vi "DAQ_Initialization.vi"(4 "AO Lasers":tag="USB-6363/ao0:3", 5 "AO Z":tag="USB-6211/ao1", 6 "AO Pockels":tag="USB-6211/ao0", 7 "DO":tag="USB-6363/port0/line0:3", 8 "error in (no error)":errorcluster, 9 "Counter":tag="USB-6363/ctr0", 10 "Timing source":tag="OnboardClock", 11 "DO | Trigger":tag="/USB-6363/PFI12") -> (0 "error out":errorcluster)   [LabVIEW 2025]
uses:
  <vilib>/DAQmx/create/channels.llb/DAQmx Create Channel (CO-Pulse Generation-Time).vi
  <vilib>/DAQmx/configure/events/hardwareSignals.llb/DAQmx Export Signal (Most Signals).vi
  <vilib>/DAQmx/create/channels.llb/DAQmx Create Channel (DO-Digital Output).vi
  <vilib>/DAQmx/configure/timing.llb/DAQmx Timing (Sample Clock).vi
  <vilib>/DAQmx/configure/trigger.llb/DAQmx Start Trigger (Digital Edge).vi
  <vilib>/DAQmx/create/channels.llb/DAQmx Create Channel (AO-Voltage-Basic).vi
  <resource>/objmgr/daqmx.rc
panel:
  in  "Export_Clock":tag="/USB-6211/PFI7"
  in  "Export_Trigger":tag="/USB-6363/PFI12"
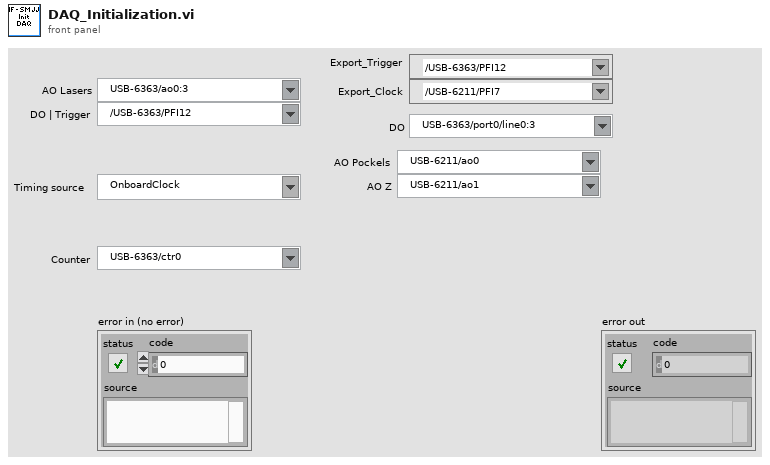
[diagram p1: front panel]
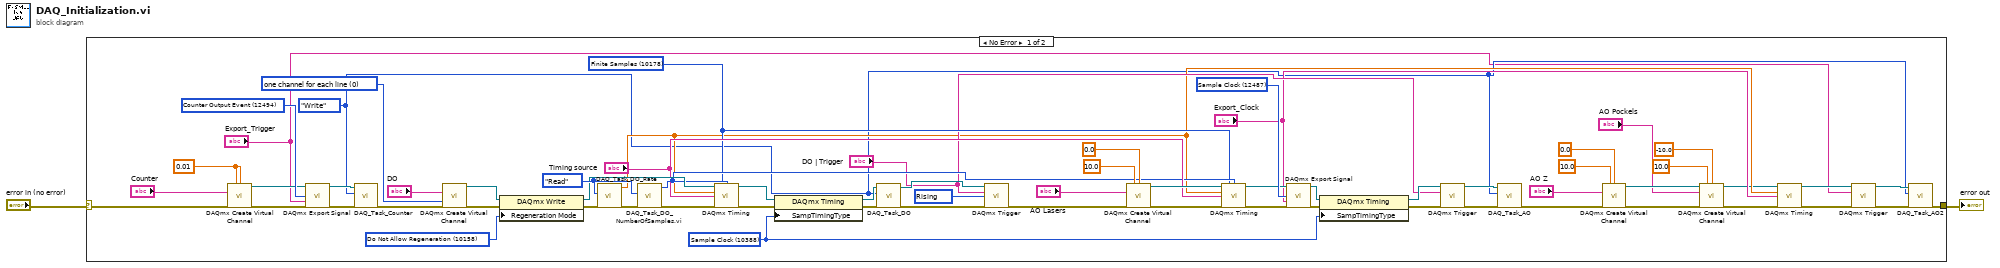
[diagram p0: block diagram]
diagram:
  n1 = case shown="No Error" "error in (no error)" {
    selector: "error in (no error)" -> [w48 w69]
    tunnel: [w12 w69] -> w1
    frame No Error {
      w25 = 12487 items=["AI Convert Clock"=12484, "10MHz Reference Clock"=12536, "20MHz Timebase Clock"=12486, "Sample Clock"=12487, "Advance Trigger"=12488, "Reference Trigger"=12490, "Start Trigger"=12491, "Advance Complete Event"=12492, "AI Hold Complete Event"=12493, "Counter Output Event"=12494, "Change Detection Event"=12511, "Watchdog Timer Expired Event"=12512] ("signal")
      w30 = 12494 items=["AI Convert Clock"=12484, "10MHz Reference Clock"=12536, "20MHz Timebase Clock"=12486, "Sample Clock"=12487, "Advance Trigger"=12488, "Reference Trigger"=12490, "Start Trigger"=12491, "Advance Complete Event"=12492, "AI Hold Complete Event"=12493, "Counter Output Event"=12494, "Change Detection Event"=12511, "Watchdog Timer Expired Event"=12512] ("signal")
      w68 = 0 items=["one channel for each line", "one channel for all lines"] ("line grouping")
      w67 = enum16{"Write", "Read"}."Read" ("Action")
      w39 = 10388 items=["Sample Clock"=10388, "Burst Handshake"=12548, "Handshake"=10389, "Implicit"=10451, "On Demand"=10390, "Change Detection"=12504, "Pipelined Sample Clock"=14668] ("SampTimingType")
      w40 = 10178 items=["Finite Samples"=10178, "Continuous Samples"=10123] ("sample mode")
      w57 = 10158 items=["Allow Regeneration"=10097, "Do Not Allow Regeneration"=10158] ("RegenMode")
      w55 = 10280 items=["Rising"=10280, "Falling"=10171] ("edge")
      w54 = 0.01 ("low time")
      w14 = enum16{"Write", "Read"}."Write" ("Action")
      n2 = call-poly <vilib>:"DAQmx Create Virtual Channel.vi"("high time"=w54, "low time"=w54, "counter"="Counter", "error in"=w48) -> ("task out"=w29:refnum<k21>, "error out"=w28:errorcluster)  [unwired: 10 in]
      n3 = call-poly <vilib>:"DAQmx Export Signal.vi"("task/channels in"=w29, "signal"=w30, "output terminal"="Export_Trigger", "error in"=w28) -> ("task out"=w26:refnum<k21>, "error out"=w27:errorcluster)  [unwired: 10 in]
      n4 = call "DAQ_Task_Counter.vi"("error in"=w27, "Action"=w14, "DAQ_Task_Counter"=w26) -> ("error out"=w51:errorcluster)  [unwired: 7 in, 1 out]
      n5 = call-poly <vilib>:"DAQmx Create Virtual Channel.vi"("lines"="DO", "line grouping"=w68, "error in"=w51) -> ("task out"=w59:refnum<k21>, "error out"=w58:errorcluster)  [unwired: 11 in]
      n6 = property class="DAQmx Write"(reference=w59, error in=w58, "Regeneration Mode"=w57) -> (reference out=w56:refnum<k21>, error out=w64:errorcluster)
      n7 = call "DAQ_Task_DO_Rate.vi"("error in"=w64, "Action"=w67) -> ("error out"=w65:errorcluster, "DO_Rate"=w17:dbl)  [unwired: 8 in]
      n8 = call "DAQ_Task_DO_NumberOfSamples.vi.vi"("error in"=w65, "Action"=w67) -> ("error out"=w66:errorcluster, "Samples"=w41:u32)  [unwired: 8 in]
      n9 = call-poly <vilib>:"DAQmx Timing.vi"("task/channels in"=w56, "sample mode"=w40, "samples per channel"=w41, "rate"=w17, "source"="Timing source", "error in"=w66) -> ("task out"=w62:refnum<k21>, "error out"=w61:errorcluster)  [unwired: 8 in]
      n10 = property class="DAQmx Timing"(reference=w62, error in=w61, "SampTimingType"=w39) -> (reference out=w63:refnum<k21>, error out=w60:errorcluster)
      n11 = call "DAQ_Task_DO.vi"("error in"=w60, "Action"=w14, "DAQ_Task_DO"=w63) -> ("error out"=w53:errorcluster, "DAQ_Task_DO"=w52:refnum<k21>)  [unwired: 7 in]
      n12 = call-poly <vilib>:"DAQmx Trigger.vi"("task/channels in"=w52, "source"="DO | Trigger", "edge"=w55, "error in"=w53) -> ("error out"=w11:errorcluster)  [unwired: 10 in, 1 out]
      n13 = call-poly <vilib>:"DAQmx Create Virtual Channel.vi"("maximum value"=10.0, "minimum value"=0.0, "physical channels"="AO Lasers", "error in"=w11) -> ("task out"=w44:refnum<k21>, "error out"=w42:errorcluster)  [unwired: 10 in]
      n14 = call-poly <vilib>:"DAQmx Timing.vi"("task/channels in"=w44, "sample mode"=w40, "samples per channel"=w41, "rate"=w17, "source"="Timing source", "error in"=w42) -> ("task out"=w24:refnum<k21>, "error out"=w23:errorcluster)  [unwired: 8 in]
      n15 = call-poly <vilib>:"DAQmx Export Signal.vi"("task/channels in"=w24, "signal"=w25, "output terminal"="Export_Clock", "error in"=w23) -> ("task out"=w21:refnum<k21>, "error out"=w22:errorcluster)  [unwired: 10 in]
      n16 = property class="DAQmx Timing"(reference=w21, error in=w22, "SampTimingType"=w39) -> (reference out=w38:refnum<k21>, error out=w37:errorcluster)
      n17 = call-poly <vilib>:"DAQmx Trigger.vi"("task/channels in"=w38, "source"="DO | Trigger", "error in"=w37) -> ("task out"=w35:refnum<k21>, "error out"=w34:errorcluster)  [unwired: 11 in]
      n18 = call "DAQ_Task_AO.vi"("error in"=w34, "Action"=w14, "DAQ_Task_DO"=w35) -> ("error out"=w20:errorcluster)  [unwired: 7 in, 1 out]
      n19 = call-poly <vilib>:"DAQmx Create Virtual Channel.vi"("maximum value"=10.0, "minimum value"=0.0, "physical channels"="AO Z", "error in"=w20) -> ("task out"=w9:refnum<k21>, "error out"=w10:errorcluster)  [unwired: 10 in]
      n20 = call-poly <vilib>:"DAQmx Create Virtual Channel.vi"("task in"=w9, "maximum value"=10.0, "minimum value"=-10.0, "physical channels"="AO Pockels", "error in"=w10) -> ("task out"=w7:refnum<k21>, "error out"=w6:errorcluster)  [unwired: 9 in]
      n21 = call-poly <vilib>:"DAQmx Timing.vi"("task/channels in"=w7, "rate"=w17, "source"="Export_Clock", "error in"=w6) -> ("task out"=w18:refnum<k21>, "error out"=w19:errorcluster)  [unwired: 10 in]
      n22 = call-poly <vilib>:"DAQmx Trigger.vi"("task/channels in"=w18, "source"="Export_Trigger", "error in"=w19) -> ("task out"=w15:refnum<k21>, "error out"=w13:errorcluster)  [unwired: 11 in]
      n23 = call "DAQ_Task_AO2.vi"("error in"=w13, "Action"=w14, "DAQ_Task_AO2"=w15) -> ("error out"=w12:errorcluster)  [unwired: 7 in, 1 out]
    }
    frame Error {
    }
  }
  "error out" <- w1
